vi "LWXPS_FileScriptHistoryRename.vi"(0 "XPS Reference IN":refnum<k24>, 2 "TCL File Name":string, 3 "LabVIEW error IN":errorcluster) -> (5 "XPS Reference OUT":refnum<k24>, 6 "Returned error code":i32, 7 "XPS Error String":string, 8 "LabVIEW error OUT":errorcluster)   [LabVIEW 2014]
uses:
  D:/XPSQ8_LabView_Library/Development/Source/Dll/Newport.XPS.CommandInterface.dll
  Dll/Newport.XPS.CommandInterface.dll
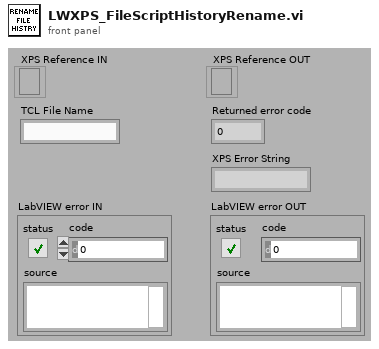
[diagram p1: front panel]
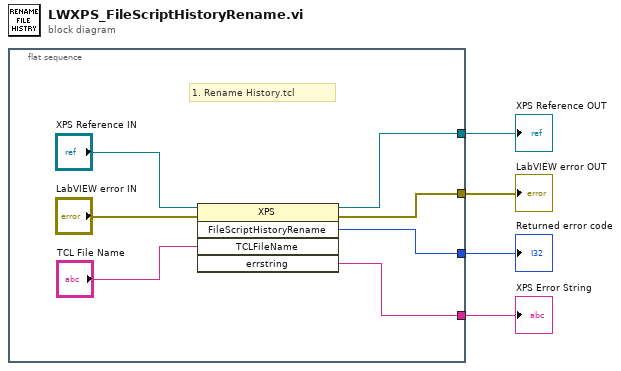
[diagram p0: block diagram]
diagram:
  n1 = flat-sequence {
    tunnel: [w5] -> w4
    tunnel: [w10] -> w3
    tunnel: [w9] -> w2
    tunnel: [w8] -> w1
    frame #0 {
      # "1. Rename History.tcl"
      n2 = invoke class="XPS" method="FileScriptHistoryRename"(reference="XPS Reference IN", error in="LabVIEW error IN", "TCLFileName"="TCL File Name") -> (reference out=w10:refnum<k24>, error out=w9:errorcluster, "FileScriptHistoryRename"=w8:i32, "errstring"=w5:string)  [unwired: 2 in, 1 out]
    }
  }
  "XPS Error String" <- w4
  "XPS Reference OUT" <- w3
  "LabVIEW error OUT" <- w2
  "Returned error code" <- w1
